vi "VFD_Host.vi"() -> ()   [LabVIEW 2017]
panel:
  in  "Control Panel Stop":bool
  in  "Pump Frequency":u16
  in  "ACTIVATE - PUMP":bool
  in  "Pump Operation Mode":i32(listbox)
  in  "TCHX Frequency":u16
  in  "ACTIVATE - TCHX":bool
  in  "TCHX Operation Mode":i32(listbox)
  in  "GS1 Stop":bool
  in  "CTAH Frequency":u16
  in  "ACTIVATE - CTAH":bool
  in  "CTAH Operation Mode":i32(listbox)
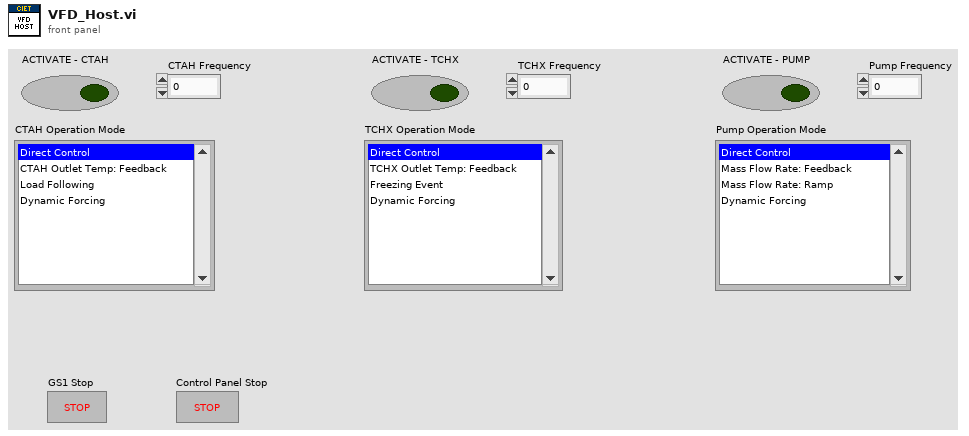
[diagram p1: front panel]
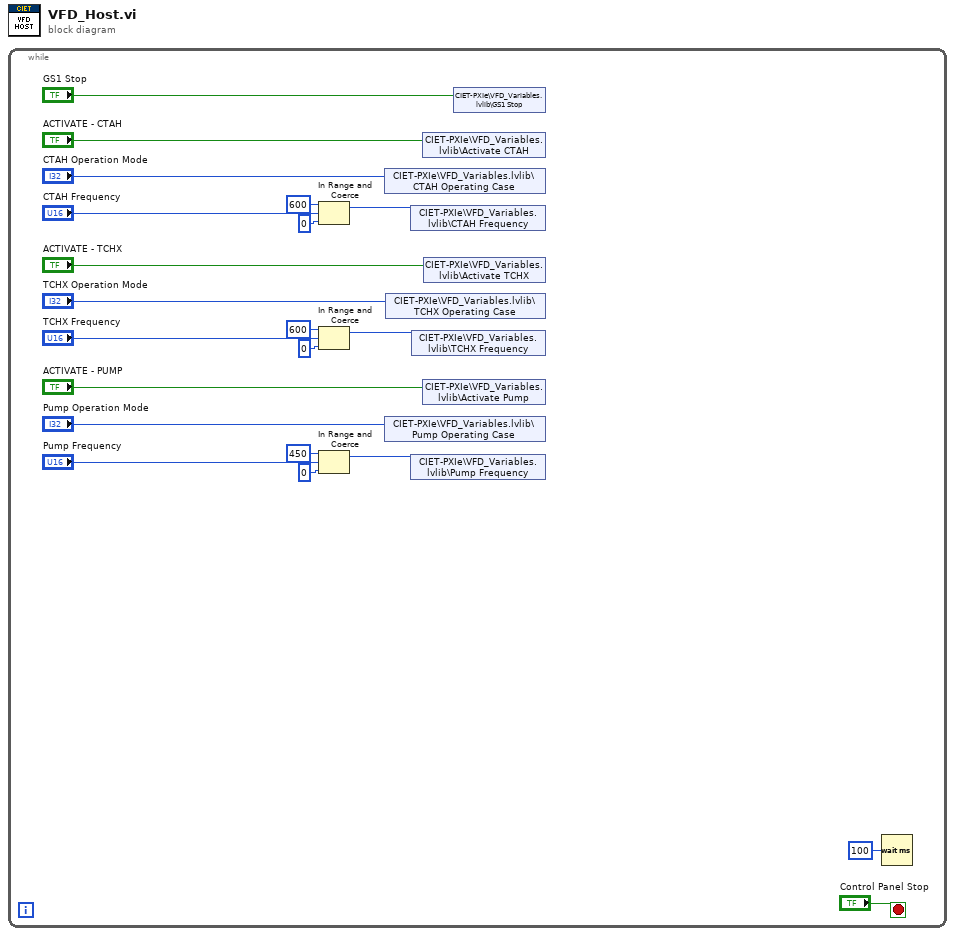
[diagram p0: block diagram]
diagram:
  n1 = while {
    stop <- "Control Panel Stop" stop-if-true
    n2 = In Range and Coerce(upper limit=u16 600, x="CTAH Frequency", lower limit=u16 0) -> (coerced(x)=w18:u16)  [unwired: 1 out]
    n3 = In Range and Coerce(upper limit=u16 600, x="TCHX Frequency", lower limit=u16 0) -> (coerced(x)=w12:u16)  [unwired: 1 out]
    n4 = In Range and Coerce(upper limit=u16 450, x="Pump Frequency", lower limit=u16 0) -> (coerced(x)=w6:u16)  [unwired: 1 out]
    n5 = shared-variable "CIET-PXIe\\VFD_Variables.lvlib\\CTAH Operating Case"("CTAH Operation Mode") -> ()  [unwired: 1 in, 1 out]
    n6 = shared-variable "CIET-PXIe\\VFD_Variables.lvlib\\Pump Operating Case"("Pump Operation Mode") -> ()  [unwired: 1 in, 1 out]
    n7 = shared-variable "CIET-PXIe\\VFD_Variables.lvlib\\TCHX Operating Case"("TCHX Operation Mode") -> ()  [unwired: 1 in, 1 out]
    n8 = shared-variable "CIET-PXIe\\VFD_Variables.lvlib\\CTAH Frequency"(w18) -> ()  [unwired: 1 in, 1 out]
    n9 = shared-variable "CIET-PXIe\\VFD_Variables.lvlib\\Pump Frequency"(w6) -> ()  [unwired: 1 in, 1 out]
    n10 = shared-variable "CIET-PXIe\\VFD_Variables.lvlib\\TCHX Frequency"(w12) -> ()  [unwired: 1 in, 1 out]
    n11 = shared-variable "CIET-PXIe\\VFD_Variables.lvlib\\Activate CTAH"("ACTIVATE - CTAH") -> ()  [unwired: 1 in, 1 out]
    n12 = shared-variable "CIET-PXIe\\VFD_Variables.lvlib\\Activate Pump"("ACTIVATE - PUMP") -> ()  [unwired: 1 in, 1 out]
    n13 = shared-variable "CIET-PXIe\\VFD_Variables.lvlib\\Activate TCHX"("ACTIVATE - TCHX") -> ()  [unwired: 1 in, 1 out]
    n14 = shared-variable "CIET-PXIe\\VFD_Variables.lvlib\\GS1 Stop"("GS1 Stop") -> ()  [unwired: 1 in, 1 out]
    n15 = Wait (ms)(milliseconds to wait=u32 100) -> ()  [unwired: 1 out]
  }
